vi "Step 1 - Design Decimation (MRate).vi"() -> ()   [LabVIEW 2023]
doc: "Demonstrates how to use the Multirate FIR Design Express VI to design a decimation filter and how to use the DFD Plot MRate Freq Response VI to analyze the characteristics of the designed filter.\n\nComplete the following steps to use this VI.\n1) Open the block diagram of the VI.\n2) Double-click the Decimation Filter Express VI to open the configuration dialog box of the Multirate FIR Design Express VI.\n<B>Note:</B> The original name of the Express VI is Multirate FIR Design. After you enter specifications in the configuration dialog box and click the <B>OK</B> button, the name of the Express VI on the block diagram changes to reflect the type of filter you design. In this example, the name changes to Decimation Filter.\n3) View the pre-defined specifications that this Express VI uses to design the decimation filter.\n4) Click the <B>OK</B> button.\n5) Run the VI.\n6) Observe the magnitude response of the designed decimation filter on the front panel."
uses:
  <vilib>/addons/Digital Filter Design/NI_DigFilterLicensed.lvlib
panel:
  out "Magnitude Response":cluster{"f0":dbl, "df":dbl, "values":dbl[]}[](graph)
  # "Select Help>>Show Context Help and move the cursor over the VI icon for more information."
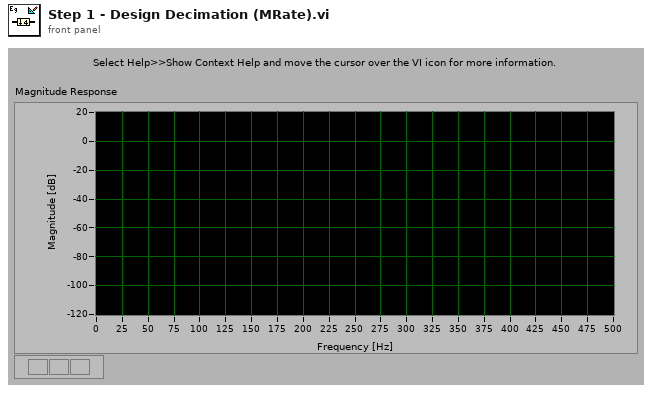
[diagram p1: front panel]
types:
  T1 = typedef "NI_DigFilterLicensed.lvlib/DFD Multirate Filter Obj.ctl" = cluster{"mMRate_Structure":enum16{"CIC", "FIR", "IIR", "Lattice"}, "mMRate_Mode":T2, "mMRate_Factor":i32, "mMRate_FIRParams":cluster{"mMRate_FIR_H":dbl[], "mMRate_FIR_IsNyquist?":bool, "mMRate_FIR_IsSymmetric?":bool}, "mMRate_CICParams":cluster{"mMRate_CIC_#Stage":i32, "mMRate_CIC_Lag":i32, "mMRate_CIC_Type":enum16{"Lowpass", "Highpass"}}, "mMRate_Order":i32, "mMRate_Version":string, "mMRate_Comments":string, "mMRate_RationalFactor":cluster{"mMRate_L":i32, "mMRate_M":i32}, "mMRate_Fs":dbl, "mMRate_Quantized?":bool, "mMRate_QFilterGain":dbl, "mMRate_CoefWl":i16, "mMRate_Scaling":cluster{"mMRate_ScaleByPowerOf2?":bool, "mMRate_ScaleType":T3}, "mMRate_InputWl":i16, "mMRate_OutputWl":i16, "mMRate_OutputMode":T4, "mMRate_MultMode":T5, "mMRate_BitPruning":bool, "mMRate_GainWl":i16, "mMRate_OutputFwl":i16, "mMRate_SumIwl":i16, "mMRate_InputIwl ":i16, "mMRate_SumWl":i16, "mMRate_CoefIwl":i16}
  T2 = typedef "NI_DigFilterLicensed.lvlib/DFD Multirate Mode.ctl" = i16
  T3 = typedef "NI_DigFilterLicensed.lvlib/DFD Coef Norm Type.ctl" = enum16{"No Norm", "Time Domain 1-Norm", "Time Domain 2-Norm", "Time Domain Inf-Norm"}
  T4 = typedef "NI_DigFilterLicensed.lvlib/DFD Round-off Mode.ctl" = enum16{"Nearest", "Truncation"}
  T5 = typedef "NI_DigFilterLicensed.lvlib/DFD FXP MRate Multiply Mode.ctl" = enum16{"Truncated", "Full"}
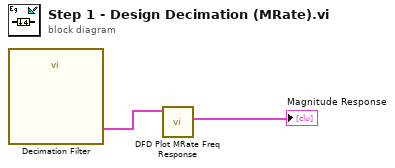
[diagram p0: block diagram]
diagram:
  n1 = call "Decimation Filter"() -> ("multirate filter out"=w1:T1)  [unwired: 11 out]
  n2 = call <vilib>:"DFD Plot MRate Freq Response.vi"("multirate filter in"=w1) -> ("magnitude response"=→"Magnitude Response":cluster{"f0":dbl, "df":dbl, "values":dbl[]}[])  [unwired: 6 in, 4 out]
